vi "Parse Files to Catagories.vi"(7 "Message Chain":string, 8 "Error in":errorcluster caption="Error in (no error)", 9 "Processed Files in":set{path}(c389), 10 "File Paths":path[](array[path]), 11 "VIDoc Parser In":refnum<class "VIDoc Parser.lvclass">) -> (0 "Error out":errorcluster, 1 "Processed Files out":set{path}(c389), 3 "VIDoc Parser Out":refnum<class "VIDoc Parser.lvclass">)   [LabVIEW 2023, in "VIDoc Parsing.lvlib" / "VIDoc Parser.lvclass"]
uses:
  VIDoc Parser.lvclass
  VIDoc Parser.lvclass/VIDoc Parser.ctl
  <vilib>/Utility/lvfile.llb/NI_FileType.lvlib
  UI Interaction/Interface/UI Interaction.lvclass
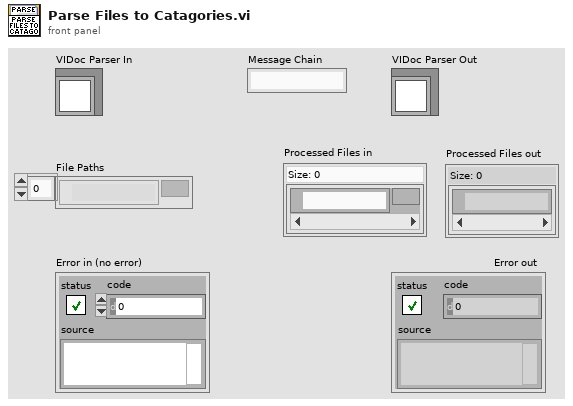
[diagram p1: front panel]
types:
  T1 = typedef "NI_FileType.lvlib/FT_FileTypes.ctl" = enum32{"Invalid file/path", "Unknown type", "Instrument", "Control", "Polymorphic VI", "Project", "Library", "LVClass", "XControl", "XNode", "CIN", "Run-time menu", "Palette menu", "LLB", "Shortcut", "Directory", "Class Private Data Control", "Statechart", "MathScript .m file", "Ladder Diagram", "LVLibp"}
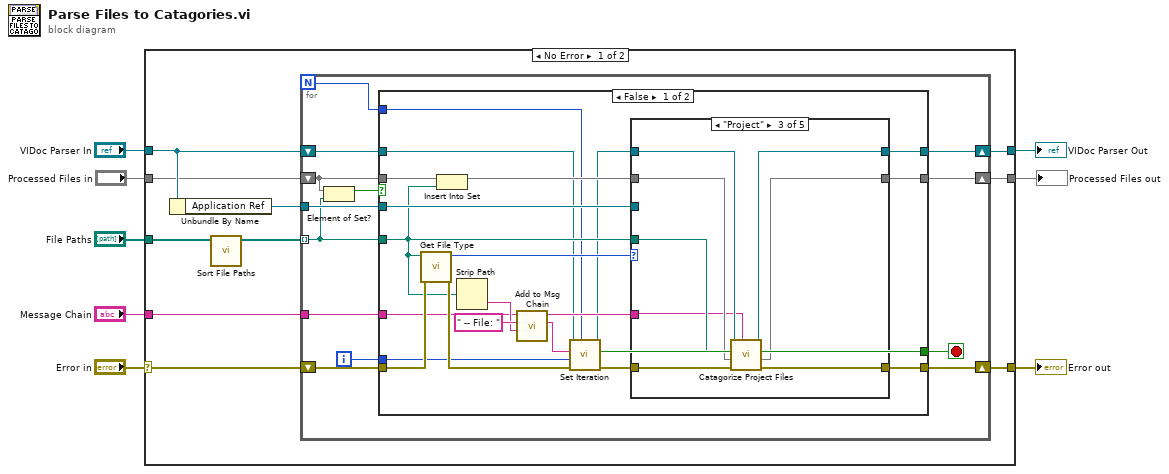
[diagram p0: block diagram]
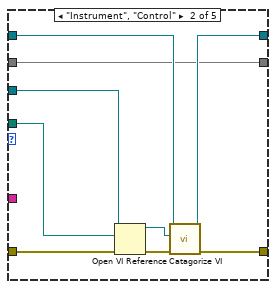
[diagram p3: hidden frame]
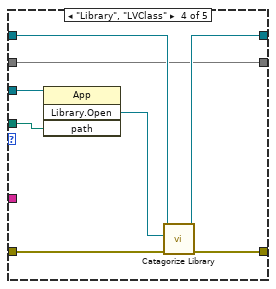
[diagram p4: hidden frame]
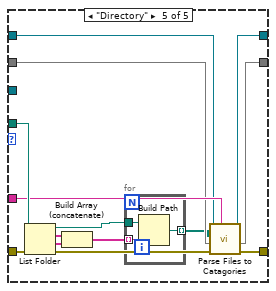
[diagram p5: hidden frame]
diagram:
  n1 = case shown="No Error" "Error in" {
    selector: "Error in" -> [w18 w102]
    tunnel: [w17 w102] -> w7
    tunnel: [w12 w101] -> w5
    tunnel: "VIDoc Parser In" -> [w16 w101]
    tunnel: "File Paths" -> [w15 _]
    tunnel: "Message Chain" -> [w14 _]
    tunnel: [w9 w100] -> w2
    tunnel: "Processed Files in" -> [w10 w100]
    frame No Error {
      n2 = Unbundle By Name(w16) -> ("Application Ref"=w13:refnum<vi>)
      n3 = call "Sort File Paths.vi"("File Paths"=w15) -> ("Sorted File Paths"=w11:path[])  [unwired: 10 in]
      n4 = for {
        N -> [w20]
        tunnel: w11 -> [w22] mode=indexing
        tunnel: w14 -> [w25]
        shift-right: [w30] -> w17
        shift-left: w18 -> [w31]
        shift-right: [w28] -> w12
        shift-left: w16 -> [w27]
        tunnel: w13 -> [w26]
        shift-right: [w24] -> w9
        shift-left: w10 -> [w23]
        i -> [w19]
        stop <- w29 stop-if-true
        n5 = Element of Set?(10:w22, 11:w23) -> (3:w21:bool)
        n6 = case shown="False" w21 {
          tunnel: w31 -> [w51 w97]
          tunnel: [w49 w97] -> w30
          tunnel: [w47 _] -> w29
          tunnel: [w43 w98] -> w28
          tunnel: w27 -> [w35 w98]
          tunnel: w26 -> [w42 _]
          tunnel: w25 -> [w41 _]
          tunnel: [w40 w99] -> w24
          tunnel: w23 -> [w39 w99]
          tunnel: w22 -> [w37 _]
          tunnel: w20 -> [w34 _]
          tunnel: w19 -> [w33 _]
          frame False {
            n7 = call <vilib>:"Get File Type.vi"("error in (no error)"=w51, "path"=w37) -> ("error out"=w50:errorcluster, "file type"=w44:T1)  [unwired: 7 in, 1 out]
            n8 = Insert Into Set(10:w37, 11:w39) -> (3:w38:set{path})  [unwired: 1 out]
            n9 = Strip Path(path=w37) -> (name=w45:string)  [unwired: 1 out]
            n10 = call "Add to Msg Chain.vi"("New"=w45, "Separator (-)"=" -- File: " ("string"), "Msg Chain in"=w41) -> ("Msg Chain out"=w32:string)  [unwired: 8 in]
            n11 = call "Set Iteration.vi"("Progress Max"=w34, "error in (no error)"=w50, "Progress Value"=w33, "Message (No Message Update)"=w32, "VIDoc Parser In"=w35) -> ("error out"=w48:errorcluster, "Abort?"=w47:bool, "VIDoc Parser Out"=w36:refnum<class "VIDoc Parser.lvclass">)  [unwired: 4 in]
            n12 = case shown="\"Project\"" w44 {
              tunnel: w37 -> [_ w58 w68 w76 w90]
              tunnel: [w54 w63 w70 w78 w91] -> w49
              tunnel: w48 -> [w54 w61 w71 w79 w93]
              tunnel: [w53 w59 w67 w74 w87] -> w43
              tunnel: w36 -> [w53 w60 w69 w75 w88]
              tunnel: w42 -> [_ w56 _ w77 _]
              tunnel: w41 -> [_ _ w64 _ w89]
              tunnel: w38 -> [w52 w55 w66 w72 w84]
              tunnel: [w52 w55 w65 w72 w83] -> w40
              frame "Invalid file/path", Default {
              }
              frame "Instrument", "Control" {
                n13 = Open VI Reference(application reference (local)=w56, vi path=w58, error in (no error)=w61) -> (vi reference=w57:refnum<vi>, error out=w62:errorcluster)  [unwired: 3 in]
                n14 = call "Catagorize VI.vi"("error in (no error)"=w62, "VI Reference"=w57, "VIDoc Parser In"=w60) -> ("error out"=w63:errorcluster, "VIDoc Parser Out"=w59:refnum<class "VIDoc Parser.lvclass">)  [unwired: 7 in]
              }
              frame "Project" {
                n15 = call "Catagorize Project Files.vi"("Message Chain"=w64, "error in (no error)"=w71, "Processed Files in"=w66, "Project File Path"=w68, "VIDoc Parser In"=w69) -> ("error out"=w70:errorcluster, "Processed Files out"=w65:set{path}, "VIDoc Parser Out"=w67:refnum<class "VIDoc Parser.lvclass">)  [unwired: 4 in]
              }
              frame "Library", "LVClass" {
                n16 = invoke class="App" method="Library.Open"(reference=w77, "path"=w76) -> ("Open Library"=w73:refnum<vi>)  [unwired: 2 in, 3 out]
                n17 = call "Catagorize Library.vi"("error in (no error)"=w79, "Library"=w73, "VIDoc Parser In"=w75) -> ("error out"=w78:errorcluster, "VIDoc Parser Out"=w74:refnum<class "VIDoc Parser.lvclass">)  [unwired: 6 in, 1 out]
              }
              frame "Directory" {
                n18 = List Folder(path=w90, error in=w93) -> (path out=w80:path, filenames=w86:string[], folder names=w85:string[], error out=w92:errorcluster)  [unwired: 2 in]
                n19 = Build Array (concatenate)(w86, w85) -> (w82:string[])
                n20 = for {
                  tunnel: w80 -> [w96]
                  tunnel: w82 -> [w95] mode=indexing
                  tunnel: [w94] -> w81 mode=indexing
                  n21 = Build Path(base path=w96, name or relative path=w95) -> (appended path=w94:path)
                }
                n22 = call "Parse Files to Catagories.vi"("Message Chain"=w89, "Error in"=w92, "Processed Files in"=w84, "File Paths"=w81, "VIDoc Parser In"=w88) -> ("Error out"=w91:errorcluster, "Processed Files out"=w83:set{path}, "VIDoc Parser Out"=w87:refnum<class "VIDoc Parser.lvclass">)  [unwired: 4 in]
              }
            }
          }
          frame True {
          }
        }
      }
    }
    frame Error {
    }
  }
  "Error out" <- w7
  "VIDoc Parser Out" <- w5
  "Processed Files out" <- w2
